vi "callpy.vi"() -> ()   [LabVIEW 2021]
panel:
  out "return value":i32
  out "error out":errorcluster
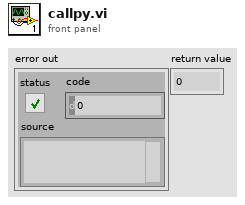
[diagram p1: front panel]
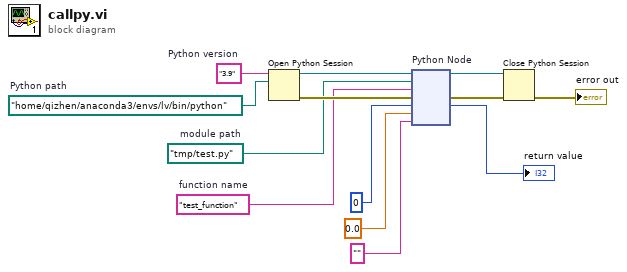
[diagram p0: block diagram]
diagram:
  w5 = "test_function"  # function name
  w6 = path "/tmp/test.py"  # module path
  w12 = path "/home/qizhen/anaconda3/envs/lv/bin/python"  # Python path
  w13 = "3.9"  # Python version
  n1 = Open Python Session(python version=w13, python path=w12) -> (session out=w11:refnum<k35>, error out=w9:errorcluster)  [unwired: 1 in]
  n2 = node "Python Node"(w11, w6, w5, w9, 0, 0.0, "") -> (w10:refnum<k35>, w8:errorcluster, →"return value":i32)  [unwired: 2 in, 2 out]
  n3 = Close Python Session(session in=w10, error in=w8) -> (11:→"error out":errorcluster)
